vi "Add Page.vi"(4 "Path":string, 5 "Pages In":refnum<k20>, 7 "Name":string, 8 "error in":errorcluster, 9 "GUID":string, 11 "Document In":refnum<k20>) -> (0 "error out":errorcluster, 3 "Document out":refnum<k20>)   [LabVIEW 2026, in "NIVS_CDEW_MetaDataObj.lvclass"]
uses:
  NIVS_CDEW_MetaDataObj.lvclass
  NIVS_CDEW_MetaDataObj.lvclass/NIVS_CDEW_MetaDataObj.ctl
  <resource>/objmgr/DOMUserDefRef.rc
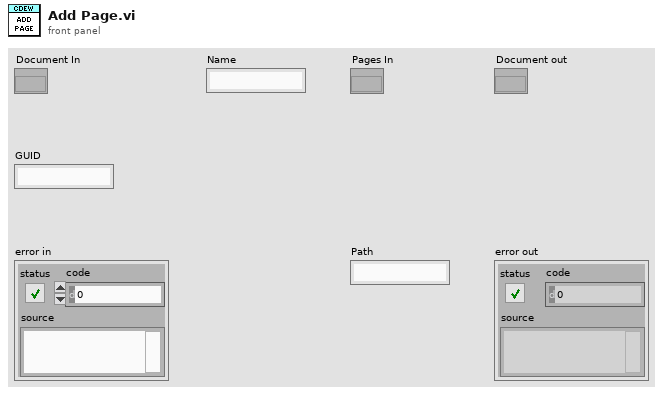
[diagram p1: front panel]
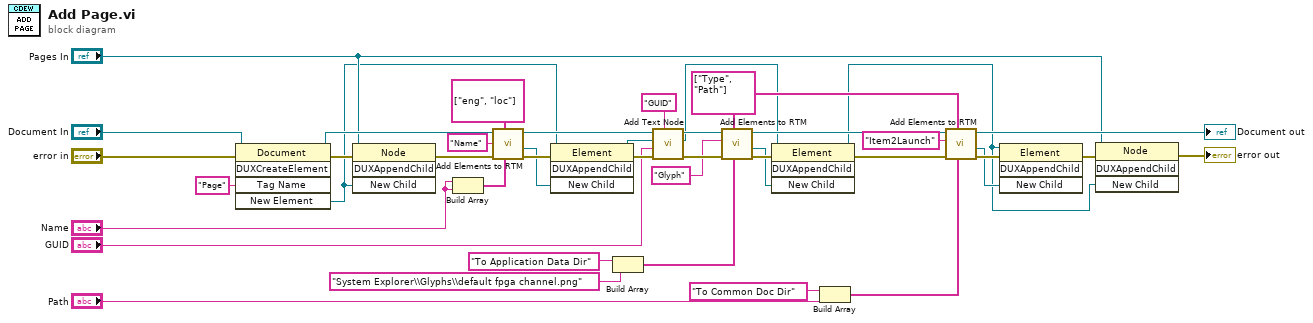
[diagram p0: block diagram]
diagram:
  w10 = string[] ["Type", "Path"]
  n1 = invoke class="Document" method="DUXCreateElement"(reference="Document In", error in="error in", "Tag Name"="Page") -> (reference out=w37:refnum<k20>, error out=w21:errorcluster, "New Element"=w2:refnum<k20>)  [unwired: 2 in, 2 out]
  n2 = invoke class="Node" method="DUXAppendChild"(reference="Pages In", error in=w21, "New Child"=w2) -> (error out=w39:errorcluster)  [unwired: 1 in, 3 out]
  n3 = Build Array("Name", "Name") -> (w33:string[])
  n4 = call "Add Elements to RTM.vi"("Tag Values"=w33, "Tag Names"=string[] ["eng", "loc"], "error in"=w39, "Element Name"="Name" ("Tag Name"), "Document In"=w37) -> ("error out"=w32:errorcluster, "Element out"=w31:refnum<k20>, "Document Out"=w19:refnum<k20>)  [unwired: 4 in]
  n5 = invoke class="Element" method="DUXAppendChild"(reference=w2, error in=w32, "New Child"=w31) -> (reference out=w18:refnum<k20>, error out=w20:errorcluster)  [unwired: 1 in, 2 out]
  n6 = Build Array("To Application Data Dir" ("Tag Data"), "System Explorer\\Glyphs\\default fpga channel.png" ("Tag Data")) -> (w7:string[])
  n7 = call "Add Text Node.vi"("Tag Name"="GUID", "error in"=w20, "Tag Data"="GUID", "Element in"=w18, "Document in"=w19) -> ("error out"=w14:errorcluster, "Element out"=w1:refnum<k20>, "Document out"=w13:refnum<k20>)  [unwired: 4 in]
  n8 = call "Add Elements to RTM.vi"("Tag Values"=w7, "Tag Names"=w10, "error in"=w14, "Element Name"="Glyph", "Document In"=w13) -> ("error out"=w6:errorcluster, "Element out"=w4:refnum<k20>, "Document Out"=w12:refnum<k20>)  [unwired: 4 in]
  n9 = invoke class="Element" method="DUXAppendChild"(reference=w1, error in=w6, "New Child"=w4) -> (reference out=w3:refnum<k20>, error out=w5:errorcluster)  [unwired: 1 in, 2 out]
  n10 = Build Array("To Common Doc Dir" ("Tag Data"), "Path") -> (w26:string[])
  n11 = call "Add Elements to RTM.vi"("Tag Values"=w26, "Tag Names"=w10, "error in"=w5, "Element Name"="Item2Launch", "Document In"=w12) -> ("error out"=w25:errorcluster, "Element out"=w24:refnum<k20>, "Document Out"=→"Document out":refnum<k20>)  [unwired: 4 in]
  n12 = invoke class="Element" method="DUXAppendChild"(reference=w3, error in=w25, "New Child"=w24) -> (error out=w23:errorcluster)  [unwired: 1 in, 3 out]
  n13 = invoke class="Node" method="DUXAppendChild"(reference="Pages In", error in=w23, "New Child"=w3) -> (error out=→"error out":errorcluster)  [unwired: 1 in, 3 out]
